vi "Lab06.vi"() -> ()   [LabVIEW 2024]
panel:
  out "AtoD":i16
  out "Temp":dbl(slide) scale=-50.0..50.0
  out "Vin, V":dbl(slide) scale=-10.0..10.0
  out "Temp Graph":dbl(graph)
  in  "stop":bool
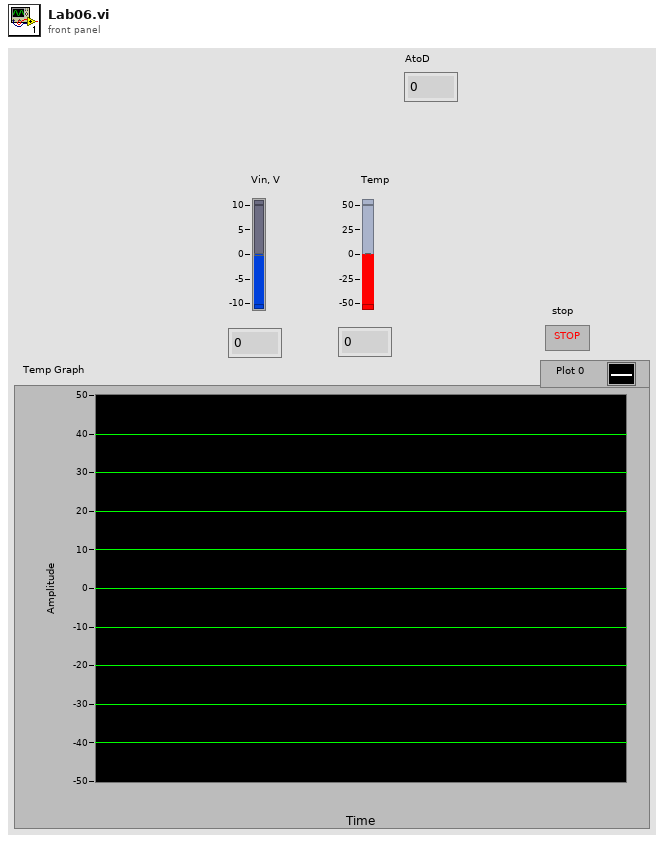
[diagram p1: front panel]
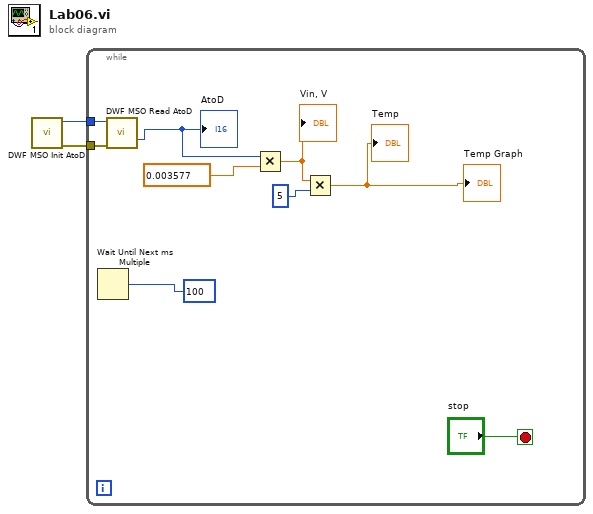
[diagram p0: block diagram]
diagram:
  n1 = call "DWF MSO Init AtoD.vi"() -> ("Error Out"=w1:errorcluster, "Instrument Handle Out"=w2:u32)  [unwired: 10 in]
  n2 = while {
    tunnel: w2 -> [w9]
    tunnel: w1 -> [w8]
    stop <- "stop" stop-if-true
    n3 = Wait Until Next ms Multiple(millisecond multiple=100) -> ()  [unwired: 1 out]
    n4 = call "DWF MSO Read AtoD.vi"("Instrument Handle In AtoD"=w9, "Error In"=w8) -> ("AtoD"=w7:i16)  [unwired: 12 in, 1 out]
    "AtoD" <- w7
    n5 = Multiply(x=w7, y=0.003577) -> (x*y=w5:dbl)
    "Vin, V" <- w5
    n6 = Multiply(x=w5, y=5) -> (x*y=→"Temp Graph" →"Temp":dbl)
  }
